vi "Load Setup File.vi"(8 "error in (no error)":errorcluster, 10 "Setup File":string, 11 "VISA resource name":refnum<visa-resource-name>) -> (0 "error out":errorcluster, 3 "VISA resource name out":refnum<visa-resource-name>)   [LabVIEW 2010, in "Temptronic TP04300.lvlib"]
doc: "This VI sends a command to TP04300 to load the setup file with the name specifed by Setup File control."
uses:
  Temptronic TP04300.lvlib
  Instance           1 23Saved   Load Setup File .vi
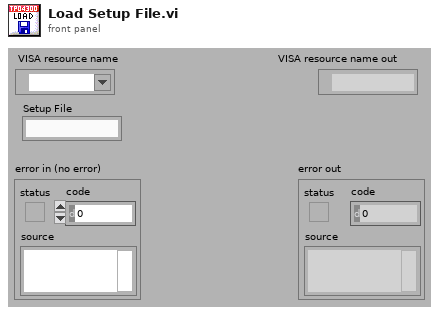
[diagram p1: front panel]
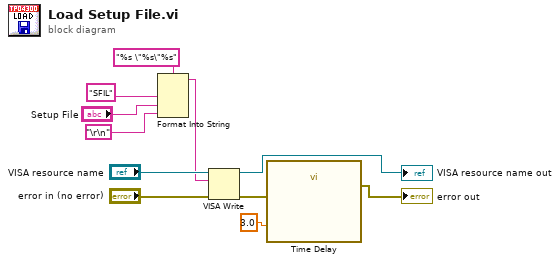
[diagram p0: block diagram]
diagram:
  n1 = Format Into String(format string="%s \"%s\"%s", "SFIL" ("format string"), "Setup File", "\r\n") -> (resulting string=w7:string)  [unwired: 2 in, 1 out]
  n2 = VISA Write(VISA resource name="VISA resource name", write buffer=w7, error in (no error)="error in (no error)") -> (VISA resource name out=→"VISA resource name out":refnum<visa-resource-name>, error out=w4:errorcluster)  [unwired: 1 out]
  n3 = call "Time Delay"("error in (no error)"=w4, "Delay Time (s)"=3.0) -> ("error out"=→"error out":errorcluster)  [unwired: 9 in]
